vi "Read Number of channels.vi"(11 "Oscilloscope in":refnum<class "Oscilloscope.lvclass">) -> (2 "Number of channels":i8=1, 3 "Oscilloscope out":refnum<class "Oscilloscope.lvclass">)   [LabVIEW 2020, in "Oscilloscope.lvclass"]
uses:
  Oscilloscope.lvclass
  Oscilloscope.lvclass/Oscilloscope.ctl
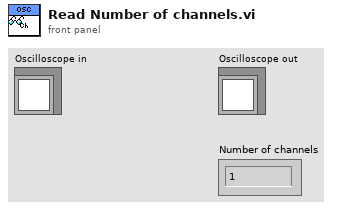
[diagram p1: front panel]
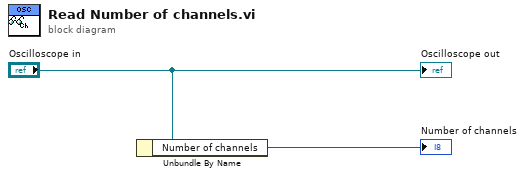
[diagram p0: block diagram]
diagram:
  n1 = Unbundle By Name("Oscilloscope in") -> ("Number of channels"=→"Number of channels":i8)
  "Oscilloscope out" <- "Oscilloscope in"
